vi "Calibrate.vi"(8 "error in (no error)":errorcluster, 11 "Instrument in":refnum<class "DMM.NI.Simulate.lvclass">) -> (0 "error out":errorcluster, 1 "Success?":bool, 2 "Result":variant, 3 "Instrument out":refnum<class "DMM.NI.Simulate.lvclass">)   [LabVIEW 2020, in "NI DMM Driver.lvlib" / "DMM.NI.Simulate.lvclass"]
doc: "Calibrate the instrument if supported. The calibration result is returned in a variant.\n\nThis implementation skips the NI DMM self calibration."
uses:
  DMM.NI.Simulate.lvclass
  NI/NI DMM Calibration Data/NI DMM Calibration Data.lvclass/NI DMM Calibration Data.ctl
  NI/NI DMM Calibration Data/NI DMM Calibration Data.lvclass
  PPL/HDH.Actor Framework.Core.Instrument Driver.lvlibp/Instrument Driver/Instrument Driver.lvclass
  C:/Current Projects/WS/PPL/HDH.Actor Framework.Core.Instrument Driver.lvlibp/Instrument Driver/Instrument Driver.lvclass
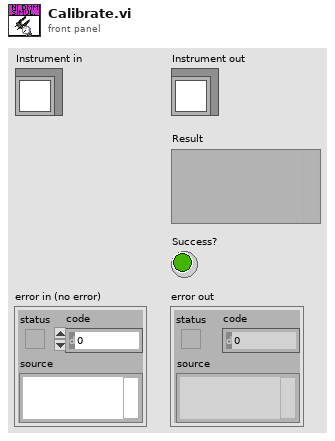
[diagram p1: front panel]
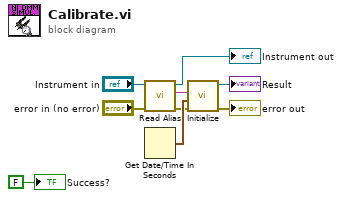
[diagram p0: block diagram]
diagram:
  n1 = call "Read Alias.vi"("error in (no error)"="error in (no error)", "Instrument in"="Instrument in") -> ("error out"=w4:errorcluster, "Alias"=w8:string, "Instrument out"=→"Instrument out":refnum<class "DMM.NI.Simulate.lvclass">)  [unwired: 7 in]
  n2 = Get Date/Time In Seconds() -> (seconds since 1Jan1904=w7:timestamp)
  n3 = call "Initialize.vi"("error in (no error)"=w4, "Time"=w7, "Alias"=w8) -> ("error out"=→"error out":errorcluster, "NI DMM Calibration Data out"=→"Result":refnum<class "NI DMM Calibration Data.lvclass">)  [unwired: 7 in]
  "Success?" <- FALSE ("Success?")
